vi "Split_and_Send.vi"(6 "rt fifo":refnum<k33>, 7 "sorted 2D array":dbl[][](array[numeric]), 9 "rt fifo 3":refnum<k33>, 10 "rt fifo 2":refnum<k33>, 11 "Byte Stream File in":refnum<file>) -> (3 "Byte Stream File out":refnum<file>)   [LabVIEW 2020]
panel:
  out "sorted 2D array 2":dbl[](array[numeric])
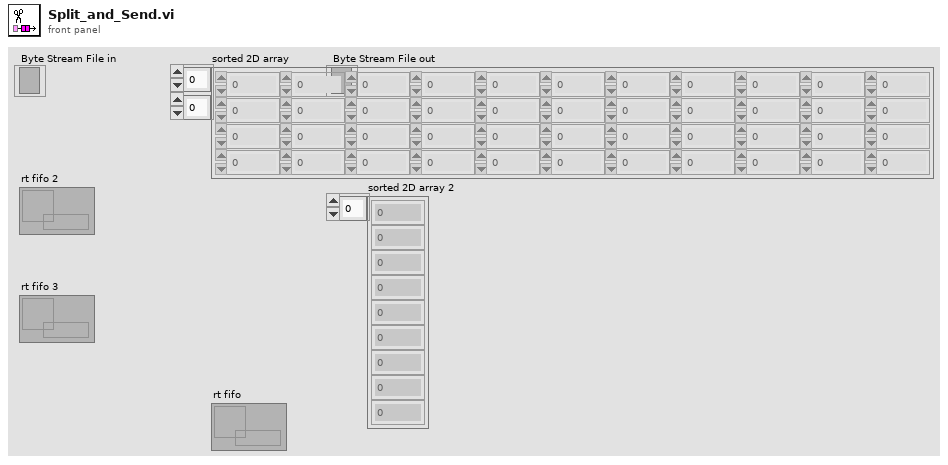
[diagram p1: front panel]
types:
  T1 = cluster{"sorted 2D array[0]":dbl, "sorted 2D array[1]":dbl, "sorted 2D array[2]":dbl, "sorted 2D array[3]":dbl, "sorted 2D array[4]":dbl, "sorted 2D array[5]":dbl, "sorted 2D array[6]":dbl, "sorted 2D array[7]":dbl, "sorted 2D array[8]":dbl}
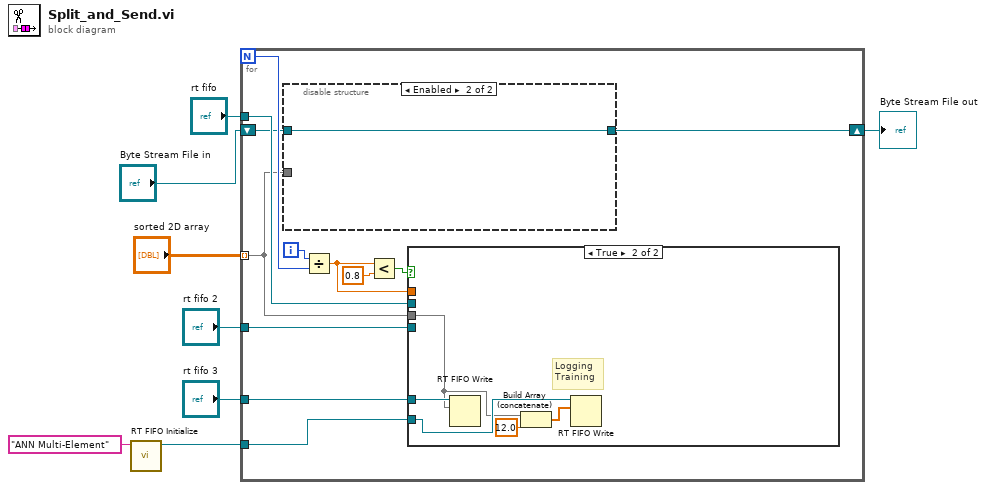
[diagram p0: block diagram]
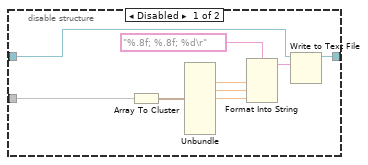
[diagram p2: hidden frame]
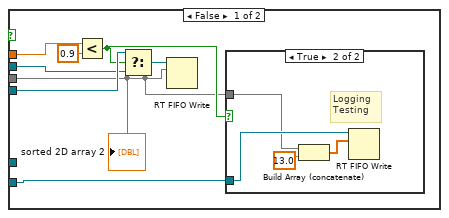
[diagram p3: hidden frame]
diagram:
  n1 = call "RT FIFO Initialize.vi"("name (unnamed)"="ANN Multi-Element") -> ("rt fifo"=w1:refnum<k33>)  [unwired: 9 in, 1 out]
  n2 = for {
    N -> [w19]
    tunnel: "rt fifo 3" -> [w15]
    tunnel: "rt fifo 2" -> [w14]
    tunnel: "rt fifo" -> [w13]
    tunnel: "sorted 2D array" -> [w10] mode=indexing
    shift-right: [w11] -> w8
    shift-left: "Byte Stream File in" -> [w12]
    tunnel: w1 -> [w9]
    i -> [w20]
    n3 = disable-structure shown="Enabled" {
      disable-tunnel: w12 -> [w29 w30]
      disable-tunnel: [w28 w30] -> w11
      disable-tunnel: w10 -> [w27 _]
      frame Disabled {
        n4 = Array To Cluster(array=w27) -> (cluster=w26:T1)
        n5 = Unbundle(w26) -> ("sorted 2D array[2]"=w25:dbl, "sorted 2D array[3]"=w24:dbl, "sorted 2D array[4]"=w23:dbl)  [unwired: 6 out]
        n6 = Format Into String(format string="%.8f; %.8f; %d\r", w25, w24, w23) -> (resulting string=w21:string)  [unwired: 2 in, 1 out]
        n7 = Write to Text File(file (use dialog)=w29, text=w21) -> (refnum out=w28:refnum<file>)  [unwired: 2 in, 2 out]
      }
      frame Enabled {
      }
    }
    n8 = Divide(x=w20, y=w19) -> (x/y=w16:dbl)
    n9 = Less?(x=w16, y=0.8) -> (x < y?=w17:bool)
    n10 = case shown="True" w17 {
      tunnel: w16 -> [w37 _]
      tunnel: w10 -> [w32 w43]
      tunnel: w15 -> [_ w47]
      tunnel: w14 -> [w36 _]
      tunnel: w13 -> [w35 _]
      tunnel: w9 -> [w31 w44]
      frame False {
        n11 = Less?(x=w37, y=0.9) -> (x < y?=w33:bool)
        n12 = Select(t=w36, s=w33, f=w35) -> (s? t:f=w34:refnum<k33>)
        n13 = RT FIFO Write(0:w34, 1:w32) -> ()  [unwired: 3 in, 4 out]
        n14 = case shown="True" w33 {
          tunnel: w32 -> [_ w40]
          tunnel: w31 -> [_ w42]
          frame False {
            # "Logging Validation"
          }
          frame True {
            # "Logging \nTesting"
            n15 = Build Array (concatenate)(w40, 13.0 ("element")) -> (w39:dbl[])
            n16 = RT FIFO Write(0:w42, 1:w39) -> ()  [unwired: 3 in, 4 out]
          }
        }
        "sorted 2D array 2" <- w32
      }
      frame True {
        # "Logging \nTraining"
        n17 = RT FIFO Write(0:w47, 1:w43) -> ()  [unwired: 3 in, 4 out]
        n18 = Build Array (concatenate)(w43, 12.0 ("element")) -> (w45:dbl[])
        n19 = RT FIFO Write(0:w44, 1:w45) -> ()  [unwired: 3 in, 4 out]
      }
    }
  }
  "Byte Stream File out" <- w8
